vi "Actor Core.vi"(8 "error in":errorcluster, 11 "UDP Link in":refnum<class "UDP Link.lvclass">) -> (0 "error out":errorcluster, 3 "Actor out":refnum<class "Actor.lvclass">)   [LabVIEW 2016, in "Assert API Components.lvlib" / "Assert Service.lvlib" / "UDP Link.lvlib" / "UDP Link.lvclass"]
doc: "(<B>Filename</B>: Actor Framework.lvlib:Actor.lvclass:Actor Core.vi)\n\nReceives messages to the actor, reacts to them, and initiates any error handling that may shut the actor down.\n\nDescendant classes may override this VI to append parallel tasks for the actor to complete while it handles messages. Overrides use the Call Parent Method node."
uses:
  UDP Link.lvclass
  <vilib>/ActorFramework/Actor/Actor.lvclass
  Base UI Actor/Base UI Actor/Base UI Actor.lvclass
  C:/Users/ukhornp/Documents/Work/Projects/actor_assert_api/Core/Base UI Actor/Base UI Actor/Base UI Actor.lvclass
  C:/Program Files (x86)/National Instruments/LabVIEW 2016/vi.lib/ActorFramework/Actor/Actor.lvclass
  <vilib>/ActorFramework/Stop Msg/Stop Msg.lvclass
  Assert Service Messages/Link Message Msg/Link Message Msg.lvclass
  <vilib>/NI/STM/TCP/Get Connection Reference (TCP).vi
  <vilib>/NI/STM/TCP/Read Message (TCP).vi
  <vilib>/NI/STM/TCP/Read Meta Data (TCP Ref).vi
panel:
  out "Iteration Count":i32
  out "data string":string
  out "IP Address":string
  out "Port Number":u16
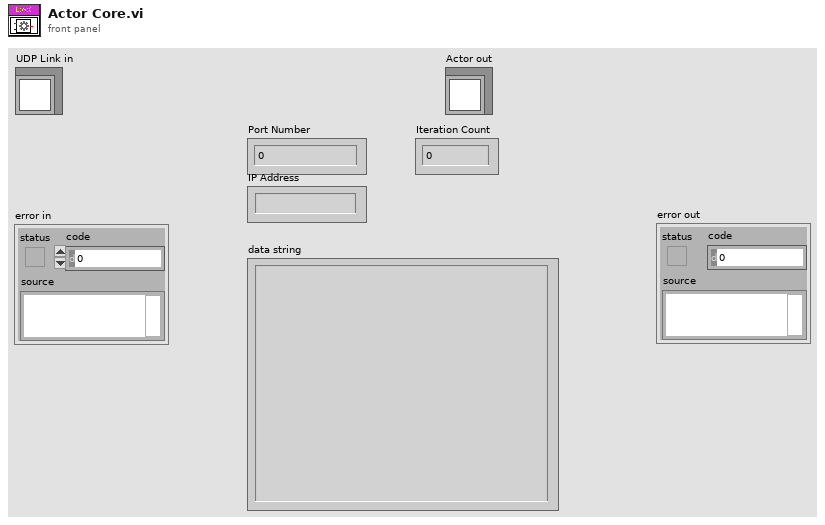
[diagram p1: front panel]
types:
  T1 = typedef "NI STM.lvlib/TCP Connection Info.ctl" = cluster{"connection ID":refnum<k5>, "meta data":T2[]}
  T2 = typedef "NI STM.lvlib/MetaDataElement.ctl" = string
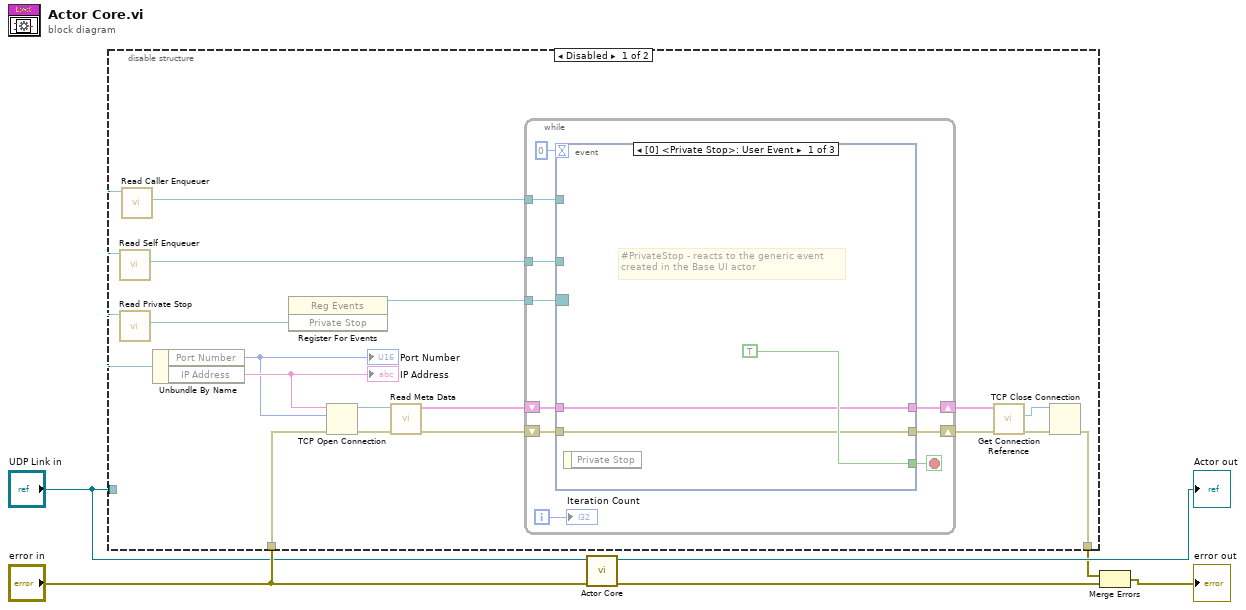
[diagram p0: block diagram]
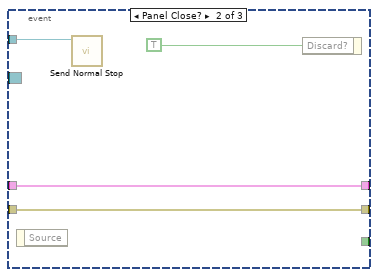
[diagram p2: hidden frame]
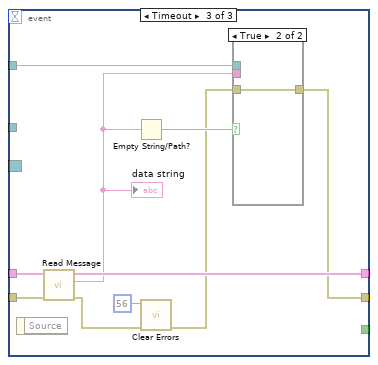
[diagram p3: hidden frame]
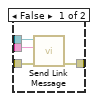
[diagram p4: hidden frame]
diagram:
  n1 = disable-structure shown="Disabled" {
    disable-tunnel: "error in" -> [w20 _]
    disable-tunnel: [w11 _] -> w2
    disable-tunnel: "UDP Link in" -> [w8 _]
    frame Disabled {
      n2 = call <vilib>:"Read Self Enqueuer.vi"("Actor"=w8) -> ("Self Enqueuer"=w23:refnum<class "Message Enqueuer.lvclass">)  [unwired: 10 in]
      n3 = call "Read Private Stop.vi"("Base UI Actor in"=w8) -> ("Private Stop"=w22:refnum<user-event>)  [unwired: 10 in]
      n4 = call <vilib>:"Read Caller Enqueuer.vi"("Actor"=w8) -> ("Caller Enqueuer"=w7:refnum<class "Message Enqueuer.lvclass">)  [unwired: 10 in]
      n5 = Unbundle By Name(w8) -> ("Port Number"=w9:u16, "IP Address"=w10:string)
      "Port Number" <- w9
      "IP Address" <- w10
      n6 = register-events(w22) -> (reference out=w21:refnum<event-registration>)  [unwired: 2 in, 1 out]
      n7 = TCP Open Connection(address=w10, remote port or service name=w9, error in (no error)=w20) -> (connection ID=w19:refnum<k5>, error out=w18:errorcluster)  [unwired: 2 in]
      n8 = call-poly <vilib>:"Read Meta Data.vi"("error in"=w18, "connection ID"=w19) -> ("error out"=w16:errorcluster, "connection info out"=w17:T1)  [unwired: 7 in, 1 out]
      n9 = while {
        tunnel: w23 -> [w33]
        tunnel: w21 -> [w32]
        shift-right: [w26] -> w13
        shift-left: w16 -> [w28]
        shift-right: [w27] -> w14
        shift-left: w17 -> [w29]
        tunnel: w7 -> [w25]
        i -> [w24]
        stop <- w31 stop-if-true
        n10 = event shown="[0] <Private Stop>: User Event" {
          selector: w32 -> [_ _ _]
          dyn-events: _ -> [_ _ _]
          timeout: 0 -> [_ _ _]
          tunnel: w33 -> [_ w39 _]
          tunnel: [TRUE _ _] -> w31
          tunnel: w29 -> [w35 w38 w48]
          tunnel: w28 -> [w34 w37 w50]
          tunnel: [w35 w38 w47] -> w27
          tunnel: [w34 w37 w41] -> w26
          tunnel: w25 -> [_ _ w44]
          event User Event {
            # "#PrivateStop - reacts to the generic event created in the Base UI actor"
            n11 = event-data() -> ()  [unwired: 1 in, 1 out]
          }
          event Panel Close? {
            n12 = event-data() -> ()  [unwired: 1 in, 1 out]
            n13 = call <vilib>:"Send Normal Stop.vi"("Message Enqueuer"=w39) -> ()  [unwired: 10 in, 1 out]
            n14 = event-data("Discard?"=TRUE) -> ()  [unwired: 1 in, 1 out]
          }
          event Timeout {
            n15 = event-data() -> ()  [unwired: 1 in, 1 out]
            n16 = call-poly <vilib>:"Read Message.vi"("error in"=w50, "connection info in"=w48) -> ("error out"=w49:errorcluster, "data string"=w43:string, "connection info out"=w47:T1)  [unwired: 4 in, 3 out]
            "data string" <- w43
            n17 = Empty String/Path?(string/path=w43) -> (empty?=w45:bool)
            n18 = call <vilib>:"Clear Errors.vi"("error in (no error)"=w49, "specific error code to clear (0: all)"=56) -> ("error out"=w42:errorcluster)  [unwired: 4 in, 1 out]
            n19 = case shown="True" w45 {
              tunnel: w44 -> [w54 _]
              tunnel: w43 -> [w53 _]
              tunnel: w42 -> [w52 w55]
              tunnel: [w51 w55] -> w41
              frame False {
                n20 = call "Send Link Message.vi"("error in (no error)"=w52, "data string"=w53, "Message Enqueuer"=w54) -> ("error out"=w51:errorcluster)  [unwired: 7 in, 1 out]
              }
              frame True {
              }
            }
          }
        }
        "Iteration Count" <- w24
      }
      n21 = call-poly <vilib>:"Get Connection Reference.vi"("error in"=w13, "connection info in"=w14) -> ("error out"=w12:errorcluster, "connection ID out"=w15:refnum<k5>)  [unwired: 7 in, 1 out]
      n22 = TCP Close Connection(connection ID=w15, error in (no error)=w12) -> (error out=w11:errorcluster)  [unwired: 1 in, 1 out]
    }
    frame Enabled {
    }
  }
  n23 = call-parent "Actor Core.vi"("error in"="error in", "Actor in"="UDP Link in") -> ("error out"=w6:errorcluster, "Actor out"=→"Actor out":refnum<class "Actor.lvclass">)  [unwired: 8 in]
  n24 = Merge Errors(w2, w6) -> (→"error out":errorcluster)
